vi "Get_Indicies_for_Bad_Tracks_(101-11)-2.vi"(4 "[IN] Current index":i32=1, 5 "[IN] Indicies of subtracks for \ntransformation (resolving)":i32[](array[numeric]), 6 "[IN] Subtracks":T1(array[cluster]), 7 "[IN] Competed elonga\ntion is reconstructed?":bool) -> (0 "[OUT] Column Number":i32, 1 "[OUT] Row Number":i32, 3 "[OUT] Competed elonga\ntion is reconstructed?":bool)   [LabVIEW 2013]
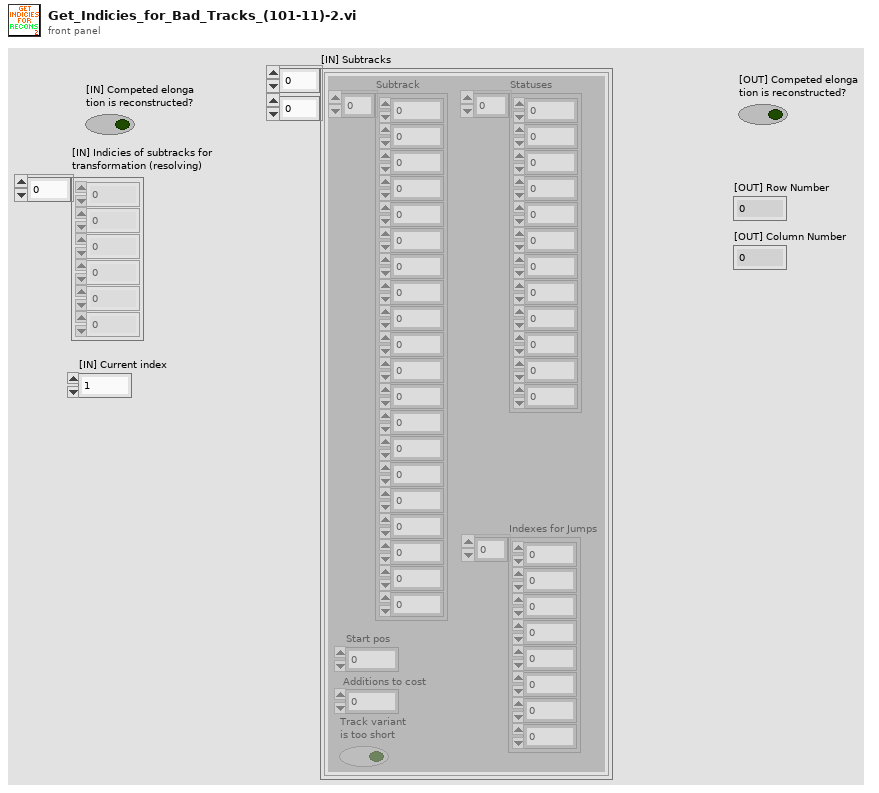
[diagram p1: front panel]
types:
  T1 = cluster{"Subtrack":dbl[], "Statuses":i16[], "Start pos":i32, "Additions to cost":i32, "Track variant \nis too short":bool, "Indexes for Jumps":i32[]}[][]
  T2 = cluster{"Subtrack":dbl[], "Statuses":i16[], "Start pos":i32, "Additions to cost":i32, "Track variant \nis too short":bool, "Indexes for Jumps":i32[]}
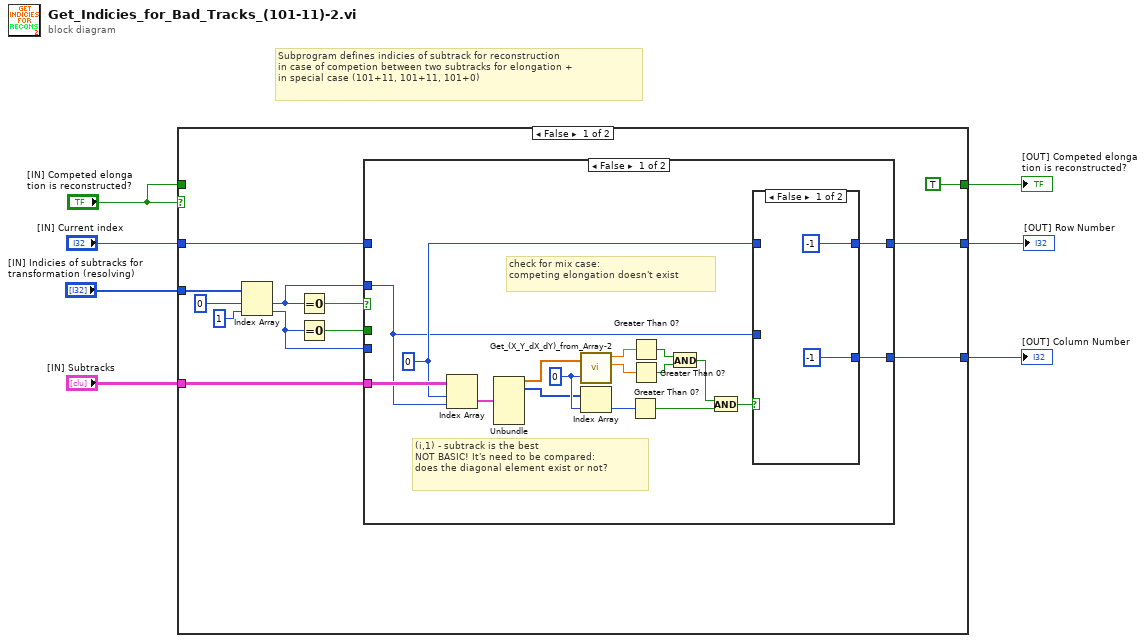
[diagram p0: block diagram]
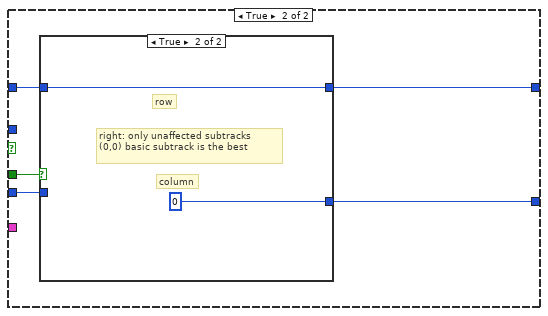
[diagram p3: hidden frame]
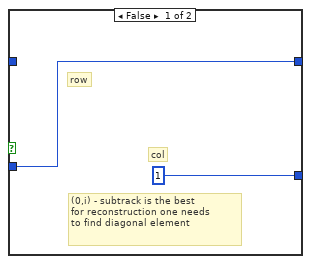
[diagram p4: hidden frame]
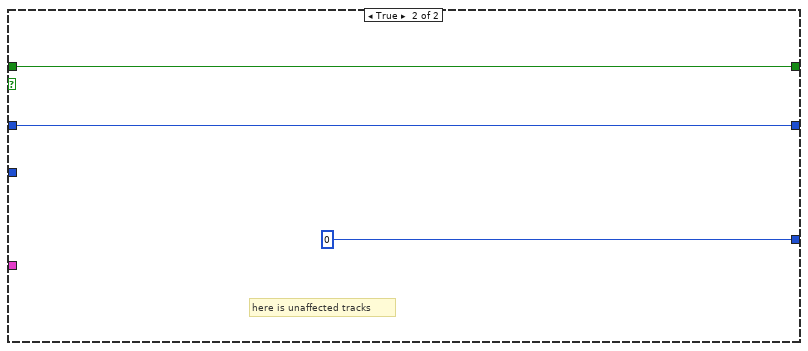
[diagram p5: hidden frame]
diagram:
  # "Subprogram defines indicies of subtrack for reconstruction\nin case of competion between two subtracks for elongation + \nin special case (101+11, 101+11, 101+0)"
  n1 = case shown="False" "[IN] Competed elonga\ntion is reconstructed?" {
    tunnel: "[IN] Indicies of subtracks for \ntransformation (resolving)" -> [w19 _]
    tunnel: "[IN] Current index" -> [w14 w51]
    tunnel: [w11 w51] -> w3
    tunnel: [w10 0 ("index")] -> w2
    tunnel: [TRUE w52] -> w5
    tunnel: "[IN] Competed elonga\ntion is reconstructed?" -> [_ w52]
    tunnel: "[IN] Subtracks" -> [w8 _]
    frame False {
      n2 = Index Array(array=w19, index #1=0 ("index"), index #2=1 ("index")) -> (element #1=w12:i32, element #2=w13:i32)
      n3 = Equal To 0?(x=w12) -> (x = 0?=w16:bool)
      n4 = Equal To 0?(x=w13) -> (x = 0?=w15:bool)
      n5 = case shown="False" w16 {
        tunnel: w15 -> [_ w45]
        tunnel: w14 -> [_ w44]
        tunnel: [w22 w43] -> w11
        tunnel: [w20 w42] -> w10
        tunnel: w13 -> [_ w41]
        tunnel: w12 -> [w21 _]
        tunnel: w8 -> [w36 _]
        frame False {
          w35 = 0
          w23 = 0 ("[IN] Current index")
          # "check for mix case:\ncompeting elongation doesn't exist"
          # "(i,1) - subtrack is the best\nNOT BASIC! It's need to be compared:\ndoes the diagonal element exist or not?"
          n6 = Index Array(array=w36, index (row)=w23, index (col)=w21) -> (element=w27:T2)
          n7 = Unbundle(w27) -> ("Subtrack"=w34:dbl[], "Statuses"=w33:i16[])  [unwired: 4 out]
          n8 = call "Get_(X_Y_dX_dY)_from_Array-2.vi"("(X,Y,dX,dY)"=w34, "Index of Displacement"=w35) -> ("X"=w31:dbl, "Y"=w30:dbl)  [unwired: 2 out]
          n9 = Index Array(array=w33, index=w35) -> (element=w28:i16)
          n10 = Greater Than 0?(x=w28) -> (x > 0?=w25:bool)
          n11 = Greater Than 0?(x=w31) -> (x > 0?=w32:bool)
          n12 = Greater Than 0?(x=w30) -> (x > 0?=w29:bool)
          n13 = And(x=w32, y=w29) -> (x .and. y?=w26:bool)
          n14 = And(x=w26, y=w25) -> (x .and. y?=w24:bool)
          n15 = case shown="False" w24 {
            tunnel: w23 -> [_ w40]
            tunnel: [-1 ("[IN] Current index") w40] -> w22
            tunnel: w21 -> [_ w39]
            tunnel: [-1 ("[IN] Current index") w39] -> w20
            frame False {
            }
            frame True {
            }
          }
        }
        frame True {
          n16 = case shown="True" w45 {
            tunnel: w44 -> [_ w49]
            tunnel: [w47 w49] -> w43
            tunnel: [1 0] -> w42
            tunnel: w41 -> [w47 _]
            frame False {
              # "(0,i) - subtrack is the best\nfor reconstruction one needs\nto find diagonal element"
              # "col"
              # "row"
            }
            frame True {
              # "right: only unaffected subtracks\n(0,0) basic subtrack is the best"
              # "column"
              # "row"
            }
          }
        }
      }
    }
    frame True {
      # "here is unaffected tracks"
    }
  }
  "[OUT] Competed elonga\ntion is reconstructed?" <- w5
  "[OUT] Row Number" <- w3
  "[OUT] Column Number" <- w2
